vi "Untitled 12.vi"() -> ()   [LabVIEW 2010]
uses:
  <vilib>/NXT/Block Support/NXT_InputPort.ctl
  <vilib>/NXT/Dual Mode Library/Sensors/Touch_Pressed.vi
  <vilib>/NXT/Dual Mode Library/Sound/Tone.vi
panel:
  in  "stop":bool
  in  "Port (Port 1)":T1 items=["Port 1", "Port 2", "Port 3", "Port 4"]
  out "Yes / No":bool
  in  "Duration (500 ms)":u16=500
  in  "Tone (440 Hz)":u16=440
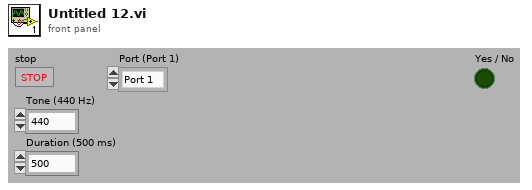
[diagram p1: front panel]
types:
  T1 = typedef "NXT_InputPort.ctl" = u8
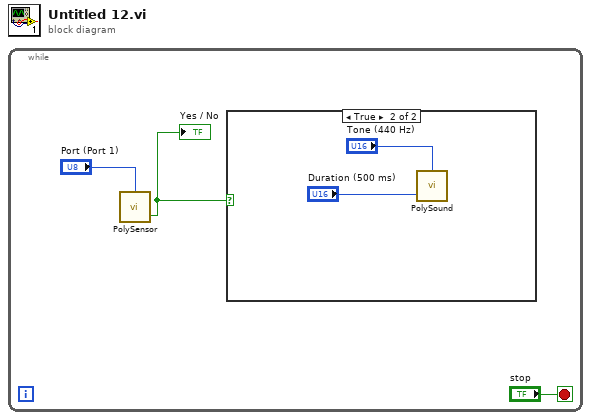
[diagram p0: block diagram]
diagram:
  n1 = while {
    stop <- "stop" stop-if-true
    n2 = call-poly <vilib>:"PolySensor.vi"("Port (Port 1)"="Port (Port 1)") -> ("Yes / No"=w3:bool)  [unwired: 2 in, 1 out]
    "Yes / No" <- w3
    n3 = case shown="True" w3 {
      frame False {
      }
      frame True {
        n4 = call-poly <vilib>:"PolySound.vi"("Duration (500 ms)"="Duration (500 ms)", "Tone (440 Hz)"="Tone (440 Hz)") -> ()  [unwired: 2 in, 1 out]
      }
    }
  }
